vi "struct_ref_T_sat_p.vi"(8 "Error (Input)":errorcluster, 10 "Saturation pressure in Pa (Input)":dbl, 11 "Reference working pair (Input)":i64) -> (0 "Error (Output)":errorcluster, 3 "Temperature in K (Output)":dbl)   [LabVIEW 2017]
doc: "ref_T_sat_p:\n * ------------\n *\n * Calculates saturation temperature in K depending on equilibrium pressure p\n * in Pa.\n *\n * Parameters:\n * -----------\n * double p_Pa:\n * Saturation pressure in Pa.\n * struct *WorkingPair:\n * Pointer of WorkingPair-struct.\n *\n * Returns:\n * --------\n * double:\n * Equilibrium temperature in K.\n *\n * History:\n * --------\n *07/13/2021, by Jannik Driesel (supervised by Mirko Engelpracht)\n * First implementation."
uses:
  data/win32bit/libsorpPropLib.dll
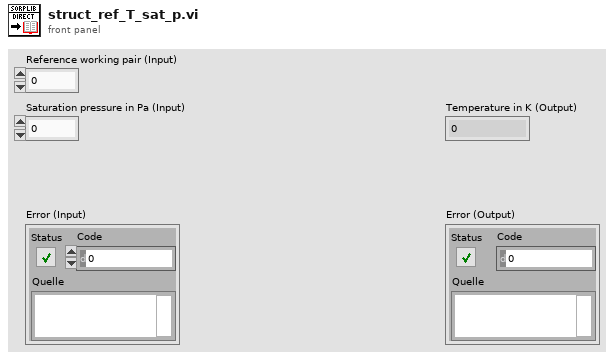
[diagram p1: front panel]
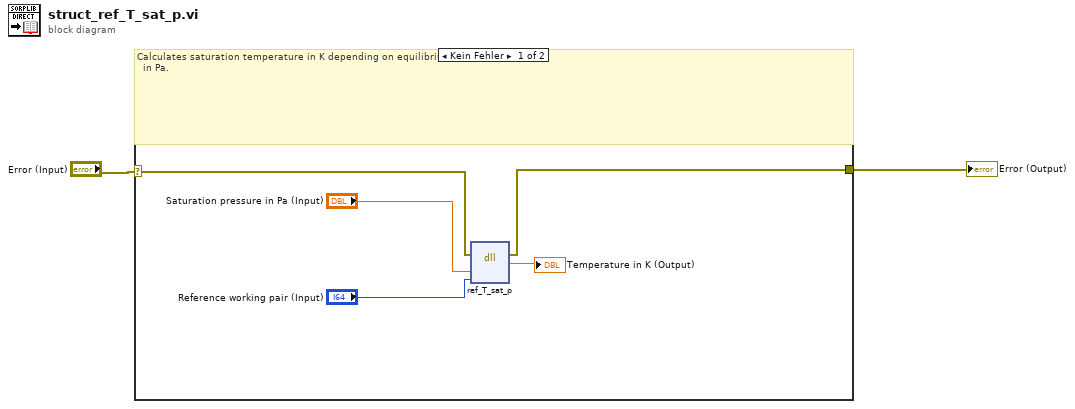
[diagram p0: block diagram]
diagram:
  n1 = case shown="Kein Fehler" "Error (Input)" {
    selector: "Error (Input)" -> [w6 w8]
    tunnel: [w7 w8] -> w2
    frame No Error {
      # "Calculates saturation temperature in K depending on equilibrium pressure p\n  in Pa."
      n2 = dll-call lib="D:/Driesel/SorpLibLocal/LabVIEW_wrapper/data/win32bit/libsorpPropLib.dll" fn="ref_T_sat_p"(error in=w6, "T_K"="Saturation pressure in Pa (Input)", "workingPair"="Reference working pair (Input)") -> (error out=w7:errorcluster, "T_sat_K"=→"Temperature in K (Output)":dbl)  [unwired: 4 in, 1 out]
    }
    frame Error {
      # "Error - No calculations"
    }
  }
  "Error (Output)" <- w2
